vi "CSB Control.vi"() -> ()   [LabVIEW 2016]
panel:
  out "Kill":bool=TRUE
  in  "X":dbl[unit](slide)
  in  "Y":dbl[unit](slide)
  in  "Z":dbl[unit](slide)
  in  "Quit":bool
  out "ID":string
  in  "URL":refnum<visa-resource-name>="tcp://localhost"
  # "CSB Control"
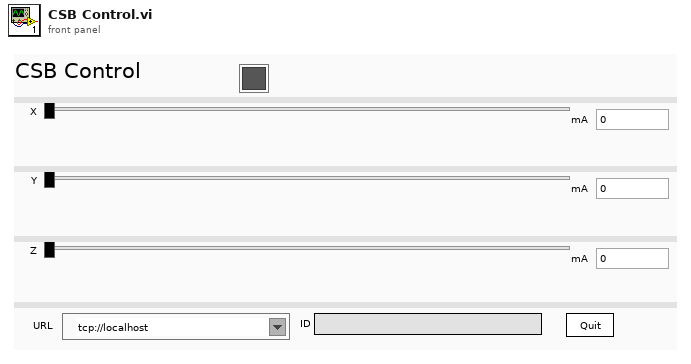
[diagram p1: front panel]
types:
  T1 = cluster{"Type":enum16{"TCP", "Serial"}, "Serial":refnum<visa-resource-name>, "TCP":refnum<k5>, "Timeout":u32}
  T2 = cluster{"Stream Description":cluster{"Stream ID":u16, "Data Type":u8, "Channels":u8, "Restart ID":u16, "Start timestamp (s)":dbl, "Sample counter":u64, "Period (s)":dbl, "Flags":u8, "Timestamp type":u8, "Name":string, "Last sample number":u64, "Last Restart ID":u16, "Version":u16, "Sample Size":u16}, "Sample #":u32, "Raw Data":string}
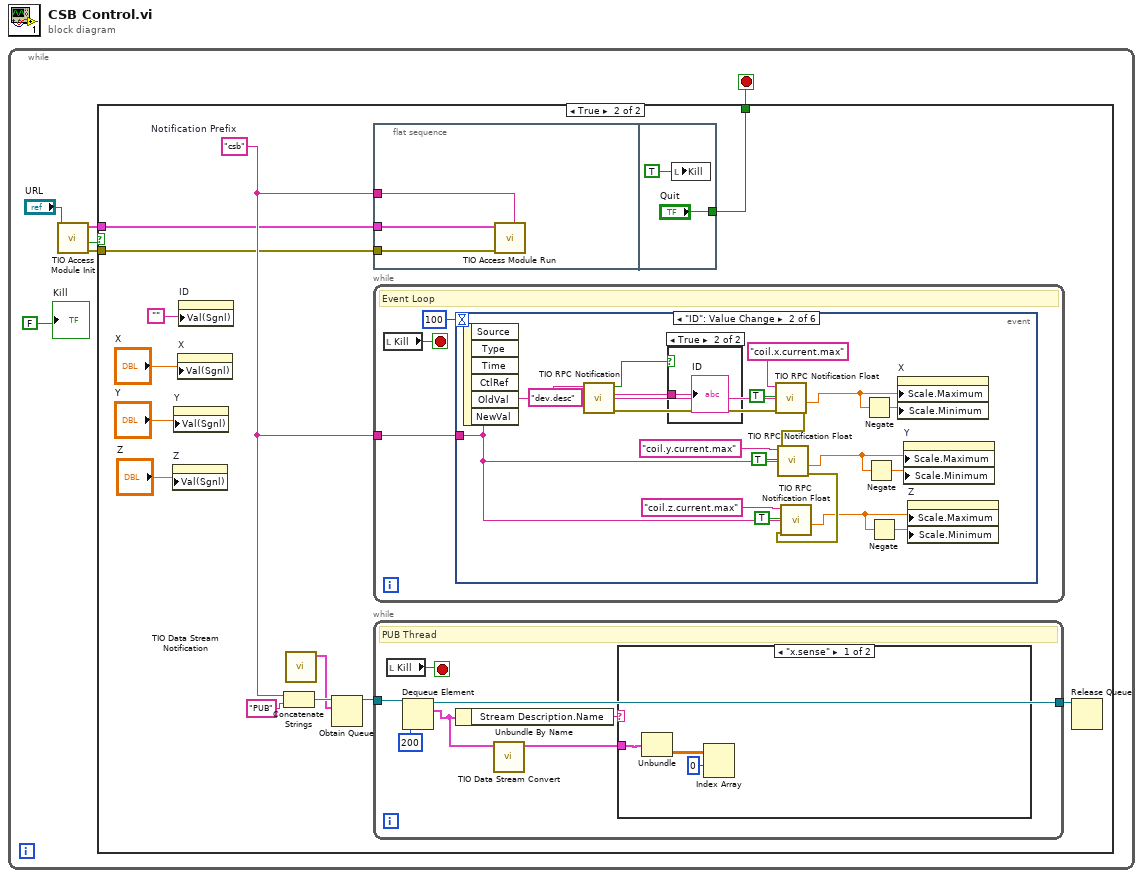
[diagram p0: block diagram]
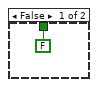
[diagram p2: hidden frame]
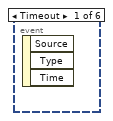
[diagram p4: hidden frame]
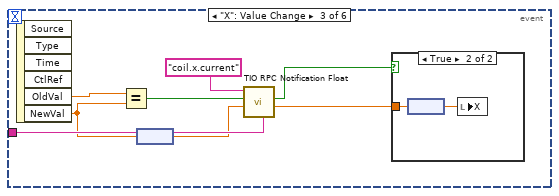
[diagram p6: hidden frame]
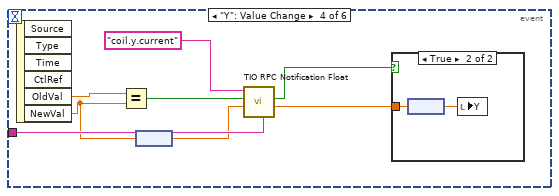
[diagram p8: hidden frame]
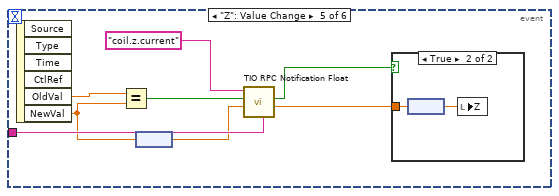
[diagram p10: hidden frame]
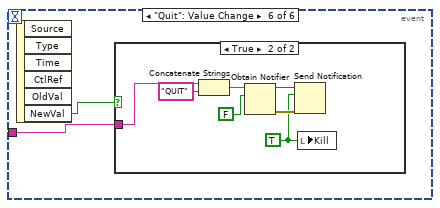
[diagram p12: hidden frame]
diagram:
  n1 = while {
    stop <- w6 stop-if-true
    n2 = call "TIO Access Module Init.vi"("URL"="URL") -> ("error out"=w3:errorcluster, "Connected"=w1:bool, "TS Connection"=w4:T1)  [unwired: 8 in]
    n3 = case shown="True" w1 {
      tunnel: [FALSE ("Quit") w13] -> w6
      tunnel: w4 -> [_ w12]
      tunnel: w3 -> [_ w11]
      frame False {
      }
      frame True {
        w14 = "csb"  # Notification Prefix
        n4 = property on="Z" class="Slide (strict)"("Val(Sgnl)"="Z") -> ()  [unwired: 2 in, 2 out]
        n5 = property on="Y" class="Slide (strict)"("Val(Sgnl)"="Y") -> ()  [unwired: 2 in, 2 out]
        n6 = property on="X" class="Slide (strict)"("Val(Sgnl)"="X") -> ()  [unwired: 2 in, 2 out]
        n7 = property on="ID" class="Str"("Val(Sgnl)"="") -> ()  [unwired: 2 in, 2 out]
        n8 = Concatenate Strings(w14, "PUB" ("name (unnamed)")) -> (w19:string)
        n9 = call "TIO Data Stream Notification.vi"() -> ("Data Stream Notification"=w15:T2)  [unwired: 11 in]
        n10 = Obtain Queue(name (unnamed)=w19, element data type=w15) -> (queue out=w17:refnum<queue>)  [unwired: 3 in, 2 out]
        n11 = flat-sequence {
          tunnel: w14 -> [w33]
          tunnel: w12 -> [w32]
          tunnel: w11 -> [w31]
          tunnel: ["Quit"] -> w13
          frame #0 {
            n12 = call "TIO Access Module Run.vi"("Notification Prefix"=w33, "error in (no error)"=w31, "TS Connection"=w32) -> ()  [unwired: 9 in]
          }
          frame #1 {
            n13 = local write "Kill"(TRUE ("Kill")) -> ()
          }
        }
        n14 = while {
          tunnel: w14 -> [w36]
          stop <- w38 stop-if-true
          # "Event Loop"
          n15 = local read "Kill"() -> (w38:bool)
          n16 = event shown="[1] \"ID\": Value Change" {
            selector: _ -> [_ _ _ _ _ _]
            dyn-events: _ -> [_ _ _ _ _ _]
            timeout: 100 -> [_ _ _ _ _ _]
            tunnel: w36 -> [_ w43 w64 w74 w84 w89]
            event Timeout {
              n17 = event-data() -> ()  [unwired: 1 in, 3 out]
            }
            event "ID": Value Change {
              n18 = event-data() -> ()  [unwired: 1 in, 6 out]
              n19 = call "TIO RPC Notification.vi"("Notification Prefix"=w43, "Topic"="dev.desc") -> ("error out"=w53:errorcluster, "REP"=w56:string, "Response"=w55:bool)  [unwired: 6 in]
              n20 = case shown="True" w55 {
                tunnel: w56 -> [_ w58]
                frame False {
                }
                frame True {
                  "ID" <- w58
                }
              }
              n21 = call "TIO RPC Notification Float.vi"("Notification"=w43, "error in (no error)"=w53, "Read"=TRUE, "String"="coil.x.current.max" ("Topic")) -> ("error out"=w47:errorcluster, "Get value (default if error)"=w52:sgl)  [unwired: 4 in, 1 out]
              n22 = call "TIO RPC Notification Float.vi"("Notification"=w43, "error in (no error)"=w47, "Read"=TRUE, "String"="coil.y.current.max" ("Topic")) -> ("error out"=w44:errorcluster, "Get value (default if error)"=w42:sgl)  [unwired: 4 in, 1 out]
              n23 = call "TIO RPC Notification Float.vi"("Notification"=w43, "error in (no error)"=w44, "Read"=TRUE, "String"="coil.z.current.max" ("Topic")) -> ("Get value (default if error)"=w39:sgl)  [unwired: 4 in, 2 out]
              n24 = Negate(x=w52) -> (-x=w51:sgl)
              n25 = Negate(x=w42) -> (-x=w41:sgl)
              n26 = Negate(x=w39) -> (-x=w40:sgl)
              n27 = property on="X" class="Slide (strict)"("Scale.Maximum"=w52, "Scale.Minimum"=w51) -> ()  [unwired: 2 in, 2 out]
              n28 = property on="Y" class="Slide (strict)"("Scale.Maximum"=w42, "Scale.Minimum"=w41) -> ()  [unwired: 2 in, 2 out]
              n29 = property on="Z" class="Slide (strict)"("Scale.Maximum"=w39, "Scale.Minimum"=w40) -> ()  [unwired: 2 in, 2 out]
            }
            event "X": Value Change {
              n30 = event-data() -> ("OldVal"=w60:dbl[unit], "NewVal"=w59:dbl[unit])  [unwired: 1 in, 4 out]
              n31 = Equal?(x=w60, y=w59) -> (x = y?=w65:bool)
              n32 = node(w59) -> (w63:dbl)
              n33 = call "TIO RPC Notification Float.vi"("Notification"=w64, "Set value"=w63, "Read"=w65, "String"="coil.x.current" ("Topic")) -> ("Get value (default if error)"=w62:sgl, "Response"=w61:bool)  [unwired: 4 in, 1 out]
              n34 = case shown="True" w61 {
                tunnel: w62 -> [_ w68]
                frame False {
                }
                frame True {
                  n35 = node(w68) -> (w67:sgl[unit])
                  n36 = local write "X"(w67) -> ()
                }
              }
            }
            event "Y": Value Change {
              n37 = event-data() -> ("OldVal"=w70:dbl[unit], "NewVal"=w69:dbl[unit])  [unwired: 1 in, 4 out]
              n38 = Equal?(x=w70, y=w69) -> (x = y?=w75:bool)
              n39 = node(w69) -> (w73:dbl)
              n40 = call "TIO RPC Notification Float.vi"("Notification"=w74, "Set value"=w73, "Read"=w75, "String"="coil.y.current" ("Topic")) -> ("Get value (default if error)"=w72:sgl, "Response"=w71:bool)  [unwired: 4 in, 1 out]
              n41 = case shown="True" w71 {
                tunnel: w72 -> [_ w78]
                frame False {
                }
                frame True {
                  n42 = node(w78) -> (w77:sgl[unit])
                  n43 = local write "Y"(w77) -> ()
                }
              }
            }
            event "Z": Value Change {
              n44 = event-data() -> ("OldVal"=w80:dbl[unit], "NewVal"=w79:dbl[unit])  [unwired: 1 in, 4 out]
              n45 = Equal?(x=w80, y=w79) -> (x = y?=w85:bool)
              n46 = node(w79) -> (w83:dbl)
              n47 = call "TIO RPC Notification Float.vi"("Notification"=w84, "Set value"=w83, "Read"=w85, "String"="coil.z.current" ("Topic")) -> ("Get value (default if error)"=w82:sgl, "Response"=w81:bool)  [unwired: 4 in, 1 out]
              n48 = case shown="True" w81 {
                tunnel: w82 -> [_ w88]
                frame False {
                }
                frame True {
                  n49 = node(w88) -> (w87:sgl[unit])
                  n50 = local write "Z"(w87) -> ()
                }
              }
            }
            event "Quit": Value Change {
              n51 = event-data() -> ("NewVal"=w90:bool)  [unwired: 1 in, 5 out]
              n52 = case shown="True" w90 {
                tunnel: w89 -> [_ w91]
                frame False {
                }
                frame True {
                  w92 = TRUE ("Kill")
                  n53 = Concatenate Strings(w91, "QUIT" ("name (unnamed)")) -> (w97:string)
                  n54 = Obtain Notifier(name (unnamed)=w97, notification data type=FALSE ("Connected")) -> (notifier out=w94:refnum<notifier>, error out=w95:errorcluster)  [unwired: 2 in, 1 out]
                  n55 = Send Notification(notification=w92, notifier=w94, error in (no error)=w95) -> ()  [unwired: 2 out]
                  n56 = local write "Kill"(w92) -> ()
                }
              }
            }
          }
        }
        n57 = while {
          tunnel: w17 -> [w26]
          tunnel: [w24] -> w16
          stop <- w27 stop-if-true
          # "PUB Thread"
          n58 = local read "Kill"() -> (w27:bool)
          n59 = Dequeue Element(queue=w26, timeout in ms (-1)=200) -> (queue out=w24:refnum<queue>, element=w21:T2)  [unwired: 1 in, 2 out]
          n60 = Unbundle By Name(w21) -> ("Stream Description.Name"=w23:string)
          n61 = call "TIO Data Stream Convert.vi"("Data Stream Notification"=w21) -> ("Waveform"=w22:cluster{dbl, dbl, dbl[][]})  [unwired: 10 in]
          n62 = case shown="\"x.sense\"" w23 {
            tunnel: w22 -> [w28 _]
            frame "x.sense" {
              n63 = Unbundle(w28) -> (w29:dbl[][])  [unwired: 2 out]
              n64 = Index Array(array=w29, index (row)=0 ("disabled index (col)")) -> ()  [unwired: 1 in, 1 out]
            }
            frame Default {
            }
          }
        }
        n65 = Release Queue(queue=w16) -> ()  [unwired: 2 in, 3 out]
      }
    }
    "Kill" <- FALSE ("Kill")
  }
